vi "Unselect.vi"(8 "error in (no error)":errorcluster, 11 "Shape":refnum<data-value>) -> (0 "error out":errorcluster, 2 "Shape out":refnum<class "Shape.lvclass">)   [LabVIEW 2015]
uses:
  Shape/Shape.lvclass
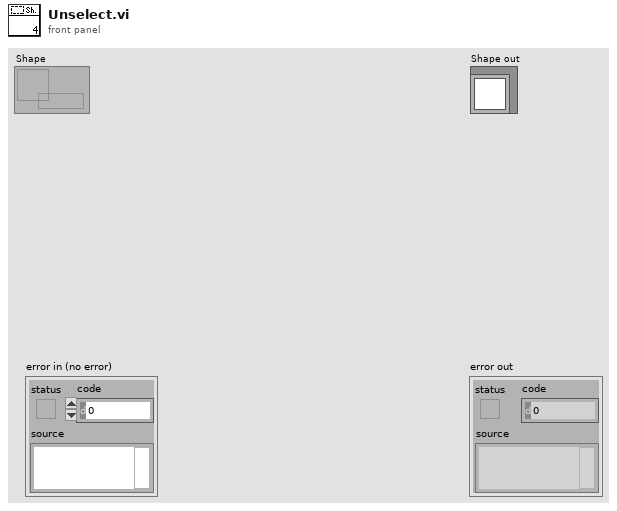
[diagram p1: front panel]
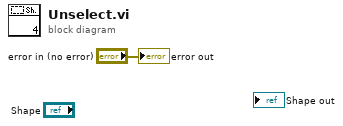
[diagram p0: block diagram]
diagram:
  "error out" <- "error in (no error)"
